vi "Configure Uncaging.vi"(6 "external trigger enabled? (Uncage ONLY)":bool, 7 "Uncage Type":T1, 9 "Gate Waveform (Digital)":digitalwaveform(waveform)={"t0"=timestamp(0 s since 1904-01-01), "dt"=0.0, "Y"={"transitions"=[], "data"=[]}, "error"={"status"=FALSE, "code"=37421928, "source"=""}}, 10 "Pockels Waveform":waveform(dbl), 11 "XY Waveform":waveform(dbl)[](array[waveform])) -> (1 "Gate Task OUT":refnum<k21>, 2 "Pockels Task OUT":refnum<k21>, 3 "XY Mirror voltage Task OUT":refnum<k21>)   [LabVIEW 2012]
uses:
  Custom Controls and Typedefs/UncageType.ctl
  modules/hyperscope modules/hyperscope subVIs/Timebase and Trigger Routing.ctl
  <vilib>/DAQmx/write.llb/DAQmx Write (Analog Wfm 1Chan NSamp).vi
  <vilib>/DAQmx/write.llb/DAQmx Write (Analog 1D Wfm NChan NSamp).vi
  <vilib>/DAQmx/write.llb/DAQmx Write (Digital 1D Wfm NChan NSamp).vi
  GFG/GFGbooleanGet.vi
  <vilib>/DAQmx/create/channels.llb/DAQmx Create Channel (AO-Voltage-Basic).vi
  <vilib>/Waveform/WDTOps.llb/WDT Number of Waveform Samples DBL.vi
  <vilib>/DAQmx/miscellaneous.llb/DAQmx Fill In Error Info.vi
  <vilib>/DAQmx/configure/trigger.llb/DAQmx Start Trigger (Digital Edge).vi
  GFG/GFGstringGet.vi
  <vilib>/DAQmx/create/channels.llb/DAQmx Create Channel (DO-Digital Output).vi
  <vilib>/Waveform/DWDTOps.llb/DWDT Digital Size.vi
  <vilib>/Waveform/DWDTOps.llb/DWDT Uncompress Digital.vi
  <resource>/objmgr/daqmx.rc
  GFG/GFG library.lvlib
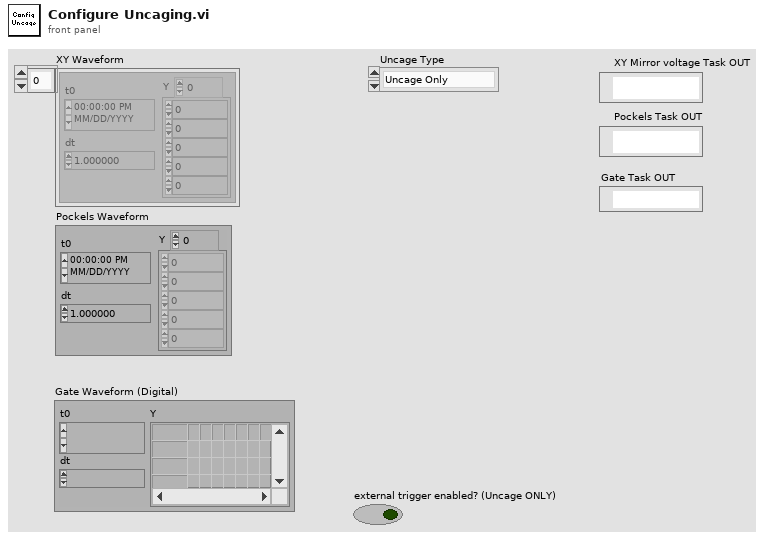
[diagram p1: front panel]
types:
  T1 = typedef "UncageType.ctl" = enum16{"Uncage Only", "Uncage & Image"}
  T2 = typedef "Timebase and Trigger Routing.ctl" = enum16{"Connect", "Disconnect all", "Disconnect Trigger"}
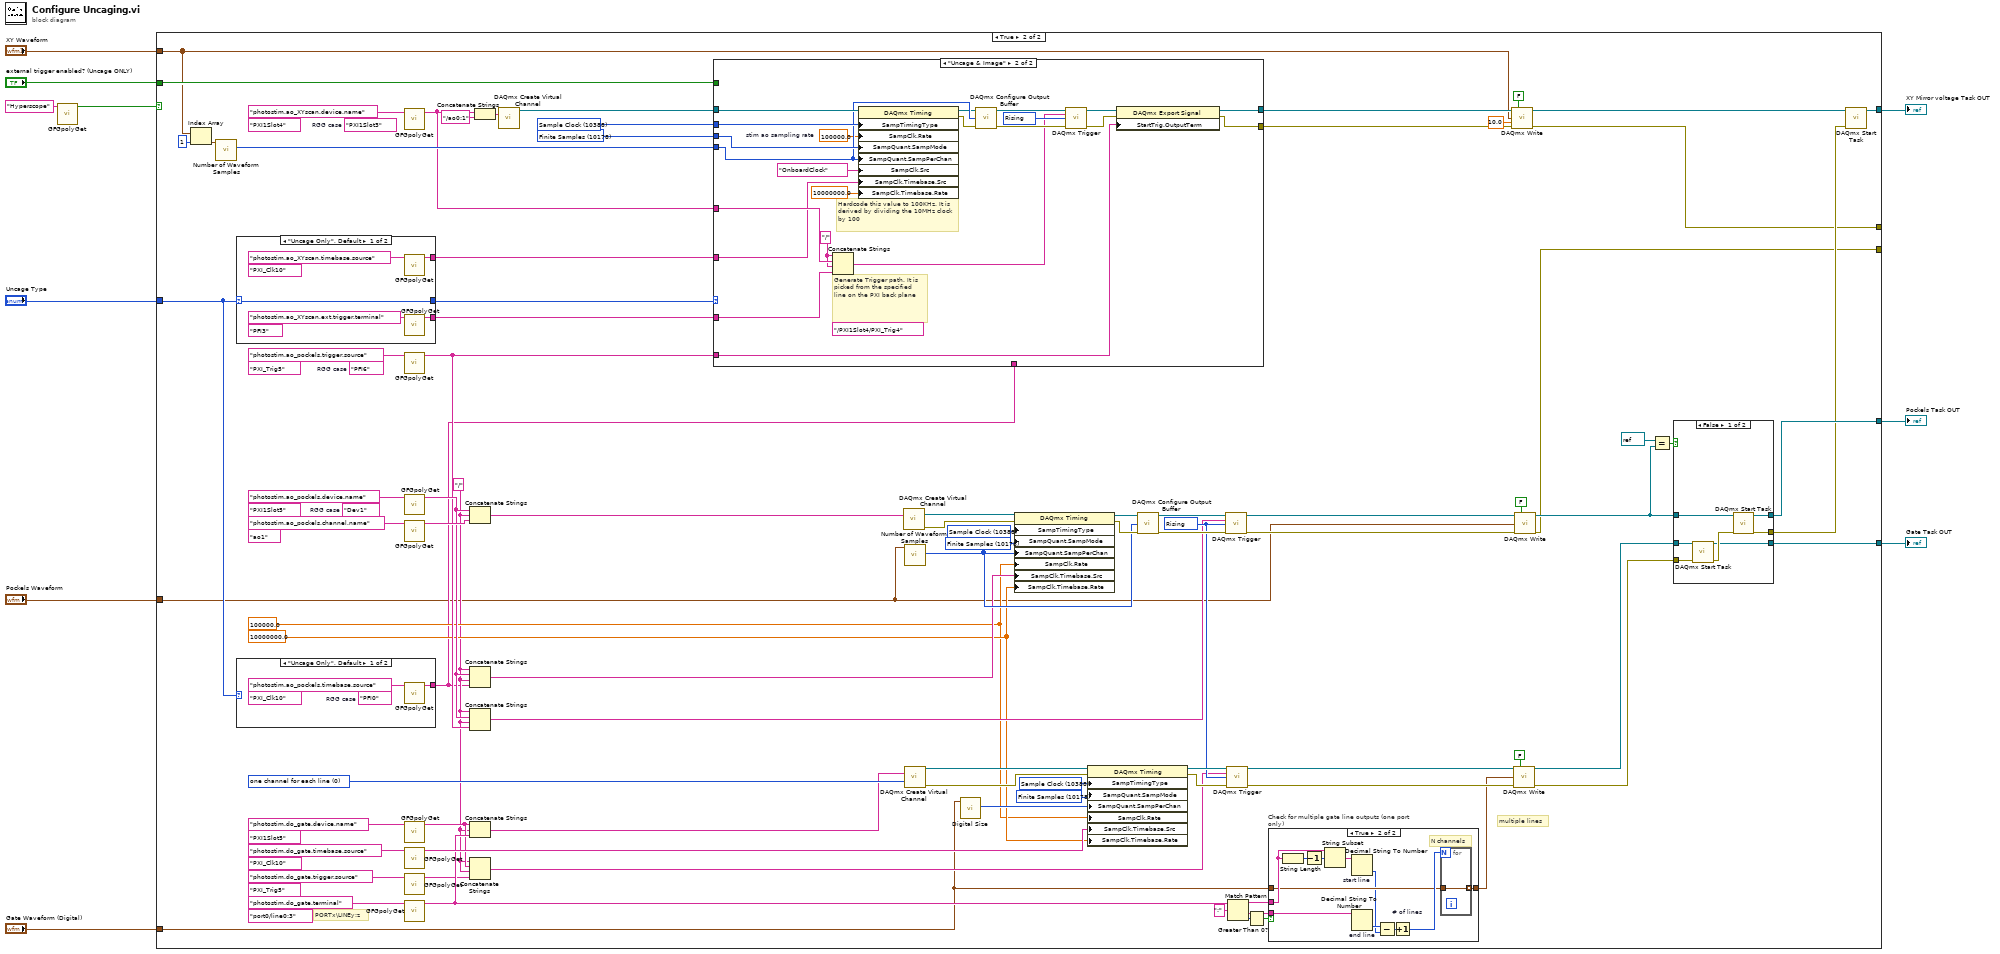
[diagram p0: block diagram]
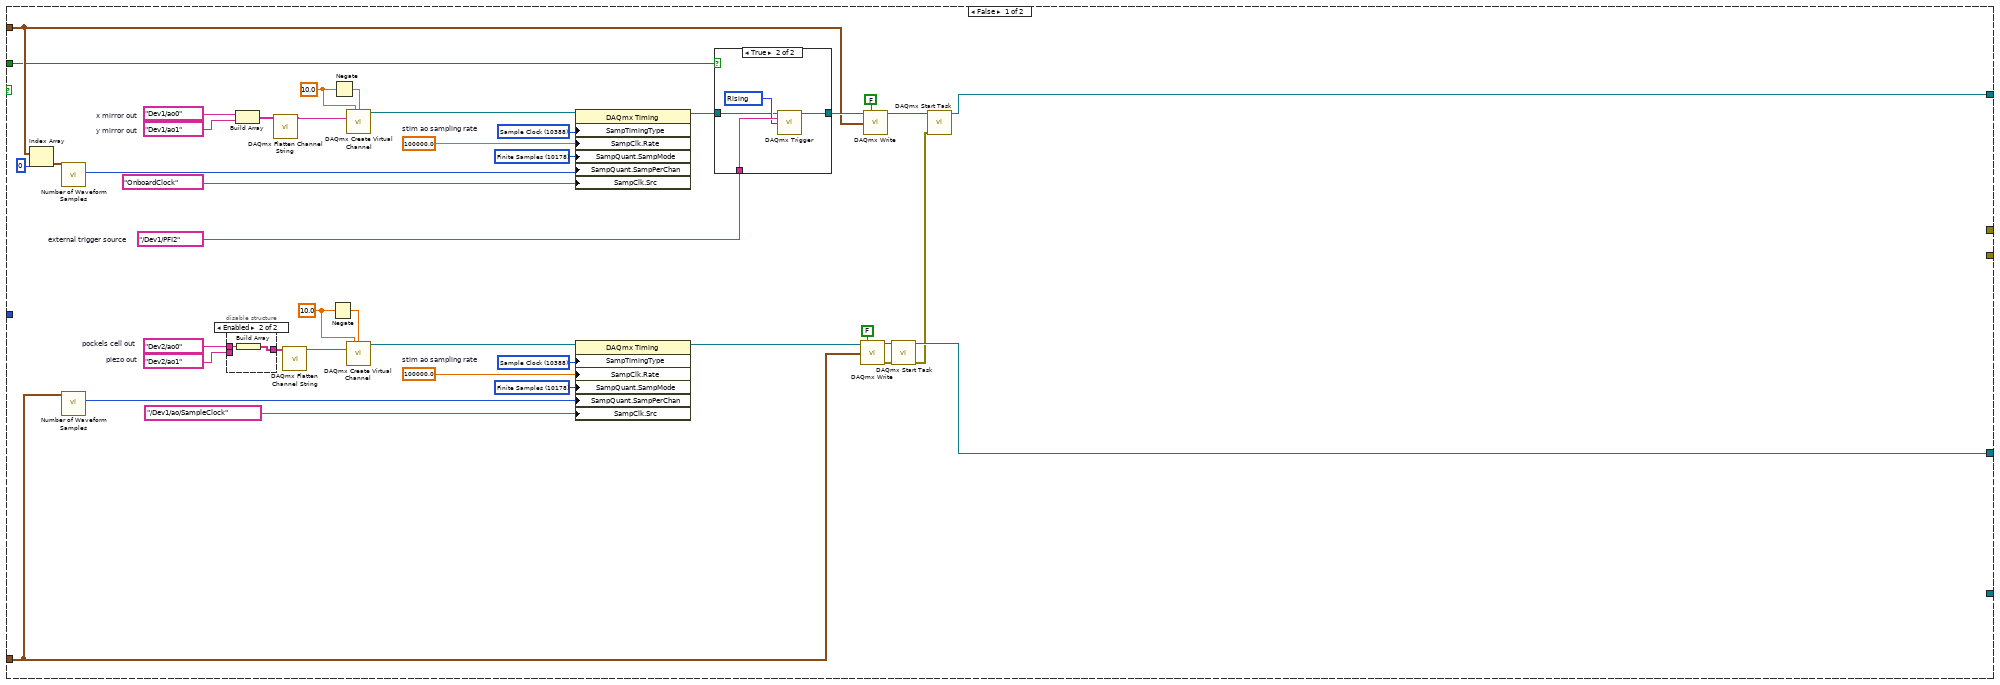
[diagram p2: hidden frame]
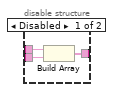
[diagram p3: hidden frame]
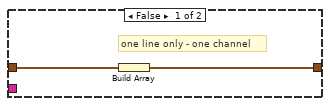
[diagram p5: hidden frame]
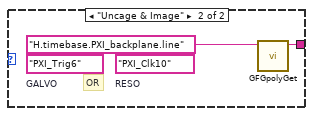
[diagram p6: hidden frame]
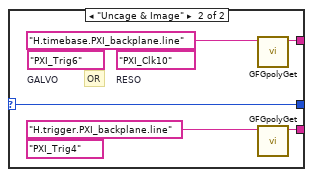
[diagram p7: hidden frame]
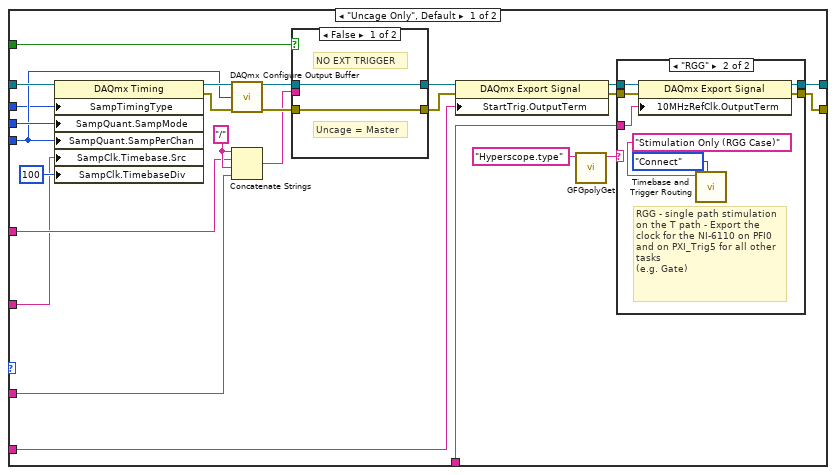
[diagram p8: hidden frame]
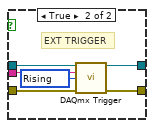
[diagram p10: hidden frame]
diagram:
  n1 = call-poly "GFGpolyGet.vi"("Variable Name in"="Hyperscope") -> ("Boolean Value OUT"=w5:bool)  [unwired: 9 in, 1 out]
  n2 = case shown="True" w5 {
    tunnel: "XY Waveform" -> [w20 w64]
    tunnel: "external trigger enabled? (Uncage ONLY)" -> [w19 w133]
    tunnel: "Uncage Type" -> [_ w121]
    tunnel: [w15 w139] -> w7
    tunnel: [w17 w138] -> w6
    tunnel: "Pockels Waveform" -> [w12 w63]
    tunnel: "Gate Waveform (Digital)" -> [_ w62]
    tunnel: [_ w124] -> w1
    tunnel: [_ w66] -> _
    tunnel: [_ w65] -> _
    frame False {
      w13 = tag "/Dev1/PFI2"  # external trigger source
      w31 = 100000.0  # stim ao sampling rate
      w30 = 100000.0  # stim ao sampling rate
      w37 = 10388 items=["Sample Clock"=10388, "Burst Handshake"=12548, "Handshake"=10389, "Implicit"=10451, "On Demand"=10390, "Change Detection"=12504, "Pipelined Sample Clock"=14668] ("SampTimingType")
      w36 = 10178 items=["Finite Samples"=10178, "Continuous Samples"=10123, "Hardware Timed Single Point"=12522] ("SampQuant.SampMode")
      w38 = 10388 items=["Sample Clock"=10388, "Burst Handshake"=12548, "Handshake"=10389, "Implicit"=10451, "On Demand"=10390, "Change Detection"=12504, "Pipelined Sample Clock"=14668] ("SampTimingType")
      w39 = 10178 items=["Finite Samples"=10178, "Continuous Samples"=10123, "Hardware Timed Single Point"=12522] ("SampQuant.SampMode")
      w42 = 10.0 ("maximum value")
      w44 = 10.0 ("maximum value")
      w46 = tag "Dev2/ao1"  # piezo out
      w47 = tag "Dev2/ao0"  # pockels cell out
      w50 = tag "Dev1/ao1"  # y mirror out
      w51 = tag "Dev1/ao0"  # x mirror out
      n3 = Index Array(array=w20, index=0) -> (element=w23:waveform(dbl))
      n4 = call-poly <vilib>:"Number of Waveform Samples.vi"("waveform in"=w23) -> ("number of samples"=w22:i32)  [unwired: 8 in, 2 out]
      n5 = call-poly <vilib>:"Number of Waveform Samples.vi"("waveform in"=w12) -> ("number of samples"=w21:i32)  [unwired: 8 in, 2 out]
      n6 = disable-structure shown="Enabled" {
        disable-tunnel: [w54 w55] -> w48
        disable-tunnel: w47 -> [w53 w56]
        disable-tunnel: w46 -> [w52 _]
        frame Disabled {
          n7 = Build Array(w53, w52) -> (w54:tag[])
        }
        frame Enabled {
          n8 = Build Array(w56) -> (w55:tag[])
        }
      }
      n9 = Build Array(w51, w50) -> (w49:tag[])
      n10 = call <vilib>:"DAQmx Flatten Channel String.vi"("names in"=w49) -> ("names out"=w43:string)  [unwired: 13 in, 1 out]
      n11 = call <vilib>:"DAQmx Flatten Channel String.vi"("names in"=w48) -> ("names out"=w40:string)  [unwired: 13 in, 1 out]
      n12 = Negate(x=w42) -> (-x=w41:dbl)
      n13 = Negate(x=w44) -> (-x=w45:dbl)
      n14 = call-poly <vilib>:"DAQmx Create Virtual Channel.vi"("maximum value"=w42, "minimum value"=w41, "physical channels"=w40) -> ("task out"=w34:refnum<k21>)  [unwired: 11 in, 1 out]
      n15 = call-poly <vilib>:"DAQmx Create Virtual Channel.vi"("maximum value"=w44, "minimum value"=w45, "physical channels"=w43) -> ("task out"=w35:refnum<k21>)  [unwired: 11 in, 1 out]
      n16 = property class="DAQmx Timing"(reference=w35, "SampTimingType"=w38, "SampClk.Rate"=w30, "SampQuant.SampMode"=w39, "SampQuant.SampPerChan"=w22, "SampClk.Src"=tag "OnboardClock") -> (reference out=w29:refnum<k21>)  [unwired: 1 in, 1 out]
      n17 = property class="DAQmx Timing"(reference=w34, "SampTimingType"=w37, "SampClk.Rate"=w31, "SampQuant.SampMode"=w36, "SampQuant.SampPerChan"=w21, "SampClk.Src"=tag "/Dev1/ao/SampleClock") -> (reference out=w25:refnum<k21>)  [unwired: 1 in, 1 out]
      n18 = case shown="True" w19 {
        tunnel: w13 -> [_ w61]
        tunnel: [w57 w60] -> w27
        tunnel: w29 -> [w57 w58]
        frame False {
        }
        frame True {
          w59 = 10280 items=["Rising"=10280, "Falling"=10171] ("edge")
          n19 = call-poly <vilib>:"DAQmx Trigger.vi"("task/channels in"=w58, "source"=w61, "edge"=w59) -> ("task out"=w60:refnum<k21>)  [unwired: 11 in, 1 out]
        }
      }
      n20 = call-poly <vilib>:"DAQmx Write.vi"("task/channels in"=w25, "auto start"=FALSE, "data"=w12) -> ("task out"=w18:refnum<k21>, "error out"=w11:errorcluster)  [unwired: 10 in, 1 out]
      n21 = call-poly <vilib>:"DAQmx Write.vi"("task/channels in"=w27, "auto start"=FALSE, "data"=w20) -> ("task out"=w16:refnum<k21>)  [unwired: 10 in, 2 out]
      n22 = call <vilib>:"DAQmx Start Task.vi"("task/channels in"=w18, "error in"=w11) -> ("task out"=w17:refnum<k21>, "error out"=w14:errorcluster)  [unwired: 12 in]
      n23 = call <vilib>:"DAQmx Start Task.vi"("task/channels in"=w16, "error in"=w14) -> ("task out"=w15:refnum<k21>)  [unwired: 12 in, 1 out]
    }
    frame True {
      (unwired) tag "Dev1"  # RGG case
      (unwired) tag "PXI1Slot3"  # RGG case
      (unwired) tag "PFI6"  # RGG case
      w69 = 100000.0 ("SampClk.Rate")
      w70 = 10000000.0 ("SampClk.Timebase.Rate")
      (unwired) tag "port0/line0:3" ("lines")
      (unwired) tag "PXI1Slot5" ("lines")
      (unwired) tag "PXI_Trig5" ("physical channels")
      w99 = 0 items=["one channel for each line", "one channel for all lines"] ("line grouping")
      (unwired) tag "PXI_Clk10" ("SampClk.Timebase.Src")
      (unwired) tag "PXI_Trig5" ("source")
      w93 = 10280 items=["Rising"=10280, "Falling"=10171] ("edge")
      w101 = 10178 items=["Finite Samples"=10178, "Continuous Samples"=10123, "Hardware Timed Single Point"=12522] ("SampQuant.SampMode")
      w102 = 10388 items=["Sample Clock"=10388, "Burst Handshake"=12548, "Handshake"=10389, "Implicit"=10451, "On Demand"=10390, "Change Detection"=12504, "Pipelined Sample Clock"=14668] ("SampTimingType")
      (unwired) tag "ao1" ("physical channels")
      w68 = "/" ("string")
      (unwired) tag "PXI1Slot5" ("physical channels")
      w120 = 10388 items=["Sample Clock"=10388, "Burst Handshake"=12548, "Handshake"=10389, "Implicit"=10451, "On Demand"=10390, "Change Detection"=12504, "Pipelined Sample Clock"=14668] ("SampTimingType")
      w119 = 10178 items=["Finite Samples"=10178, "Continuous Samples"=10123, "Hardware Timed Single Point"=12522] ("SampQuant.SampMode")
      (unwired) tag "PXI1Slot4" ("physical channels")
      w148 = 10388 items=["Sample Clock"=10388, "Burst Handshake"=12548, "Handshake"=10389, "Implicit"=10451, "On Demand"=10390, "Change Detection"=12504, "Pipelined Sample Clock"=14668] ("SampTimingType")
      w147 = 10178 items=["Finite Samples"=10178, "Continuous Samples"=10123, "Hardware Timed Single Point"=12522] ("SampQuant.SampMode")
      # "multiple lines"
      # "PORTx\\LINEy:z"
      n24 = Index Array(array=w64, index=1) -> (element=w135:waveform(dbl))
      n25 = call-poly <vilib>:"Number of Waveform Samples.vi"("waveform in"=w135) -> ("number of samples"=w134:i32)  [unwired: 8 in, 2 out]
      n26 = case shown="\"Uncage Only\", Default" w121 {
        selector: w121 -> [w169 w172]
        tunnel: [w171 w176] -> w128
        tunnel: [w167 w175] -> w127
        tunnel: [w169 w172] -> w80
        frame "Uncage Only", Default {
          (unwired) tag "PFI3"
          (unwired) tag "PXI_Clk10" ("SampClk.Timebase.Src")
          n27 = call-poly "GFGpolyGet.vi"("Variable Name in"="photostim.ao_XYscan.timebase.source") -> ("String"=w171:string)  [unwired: 9 in, 1 out]
          n28 = call-poly "GFGpolyGet.vi"("Variable Name in"="photostim.ao_XYscan.ext.trigger.terminal") -> ("String"=w167:string)  [unwired: 9 in, 1 out]
        }
        frame "Uncage & Image" {
          (unwired) tag "PXI_Clk10"  # RESO
          (unwired) tag "PXI_Trig6"  # GALVO
          (unwired) tag "PXI_Trig4" ("physical channels")
          # "OR"
          n29 = call-poly "GFGpolyGet.vi"("Variable Name in"="H.timebase.PXI_backplane.line") -> ("String"=w176:string)  [unwired: 9 in, 1 out]
          n30 = call-poly "GFGpolyGet.vi"("Variable Name in"="H.trigger.PXI_backplane.line") -> ("String"=w175:string)  [unwired: 9 in, 1 out]
        }
      }
      n31 = case shown="\"Uncage Only\", Default" w121 {
        tunnel: [w163 w165] -> w67
        frame "Uncage Only", Default {
          (unwired) tag "PFI0"  # RGG case
          (unwired) tag "PXI_Clk10" ("SampClk.Timebase.Src")
          n32 = call-poly "GFGpolyGet.vi"("Variable Name in"="photostim.ao_pockels.timebase.source") -> ("String"=w163:string)  [unwired: 9 in, 1 out]
        }
        frame "Uncage & Image" {
          (unwired) tag "PXI_Clk10"  # RESO
          (unwired) tag "PXI_Trig6"  # GALVO
          # "OR"
          n33 = call-poly "GFGpolyGet.vi"("Variable Name in"="H.timebase.PXI_backplane.line") -> ("String"=w165:string)  [unwired: 9 in, 1 out]
        }
      }
      n34 = call-poly "GFGpolyGet.vi"("Variable Name in"="photostim.ao_XYscan.device.name") -> ("String"=w129:string)  [unwired: 9 in, 1 out]
      n35 = call-poly "GFGpolyGet.vi"("Variable Name in"="photostim.ao_pockels.trigger.source") -> ("String"=w77:string)  [unwired: 9 in, 1 out]
      n36 = call-poly "GFGpolyGet.vi"("Variable Name in"="photostim.ao_pockels.device.name") -> ("String"=w104:string)  [unwired: 9 in, 1 out]
      n37 = call-poly "GFGpolyGet.vi"("Variable Name in"="photostim.ao_pockels.channel.name") -> ("String"=w111:string)  [unwired: 9 in, 1 out]
      n38 = call-poly "GFGpolyGet.vi"("Variable Name in"="photostim.do_gate.device.name") -> ("String"=w74:string)  [unwired: 9 in, 1 out]
      n39 = call-poly "GFGpolyGet.vi"("Variable Name in"="photostim.do_gate.timebase.source") -> ("String"=w90:string)  [unwired: 9 in, 1 out]
      n40 = call-poly "GFGpolyGet.vi"("Variable Name in"="photostim.do_gate.trigger.source") -> ("String"=w73:string)  [unwired: 9 in, 1 out]
      n41 = call-poly "GFGpolyGet.vi"("Variable Name in"="photostim.do_gate.terminal") -> ("String"=w82:string)  [unwired: 9 in, 1 out]
      n42 = Concatenate Strings(w104, w68, w111) -> (w110:string)
      n43 = Concatenate Strings(w68, w104, w68, w67) -> (w89:string)
      n44 = Concatenate Strings(w68, w104, w68, w77) -> (w78:string)
      n45 = Concatenate Strings(w74, w68, w82) -> (w88:string)
      n46 = Concatenate Strings(w68, w74, w68, w73) -> (w72:string)
      n47 = Concatenate Strings(w129, "/ao0:1" ("string")) -> (w130:string)
      n48 = call-poly <vilib>:"DAQmx Create Virtual Channel.vi"("physical channels"=w130) -> ("task out"=w136:refnum<k21>)  [unwired: 13 in, 1 out]
      n49 = case shown="\"Uncage & Image\"" w80 {
        tunnel: w148 -> [w190 w240]
        tunnel: w147 -> [w201 w239]
        tunnel: [w180 w237] -> w122
        tunnel: w136 -> [w200 w238]
        tunnel: w134 -> [w198 w236]
        tunnel: w133 -> [w196 _]
        tunnel: [w179 w235] -> w123
        tunnel: w129 -> [w189 w234]
        tunnel: w128 -> [w185 w233]
        tunnel: w127 -> [w183 w232]
        tunnel: w77 -> [w184 w231]
        tunnel: w67 -> [w177 _]
        frame "Uncage Only", Default {
          w192 = "/" ("string")
          n50 = property class="DAQmx Timing"(reference=w200, "SampTimingType"=w190, "SampQuant.SampMode"=w201, "SampQuant.SampPerChan"=w198, "SampClk.Timebase.Src"=w185, "SampClk.TimebaseDiv"=u32 100) -> (reference out=w199:refnum<k21>, error out=w194:errorcluster)  [unwired: 1 in]
          n51 = call <vilib>:"DAQmx Configure Output Buffer.vi"("task/channels in"=w199, "buffer size (in samples per channel)"=w198, "error in"=w194) -> ("task out"=w197:refnum<k21>, "error out"=w193:errorcluster)  [unwired: 11 in]
          n52 = Concatenate Strings(w192, w189, w192, w183) -> (w191:string)
          n53 = case shown="False" w196 {
            tunnel: w191 -> [_ w218]
            tunnel: [w212 w217] -> w187
            tunnel: w197 -> [w212 w215]
            tunnel: w193 -> [w211 w214]
            tunnel: [w211 w213] -> w188
            frame False {
              # "Uncage = Master"
              # "NO EXT TRIGGER"
            }
            frame True {
              w216 = 10280 items=["Rising"=10280, "Falling"=10171] ("edge")
              # "EXT TRIGGER"
              n54 = call-poly <vilib>:"DAQmx Trigger.vi"("task/channels in"=w215, "source"=w218, "edge"=w216, "error in"=w214) -> ("task out"=w217:refnum<k21>, "error out"=w213:errorcluster)  [unwired: 10 in]
            }
          }
          n55 = property class="DAQmx Export Signal"(reference=w187, error in=w188, "StartTrig.OutputTerm"=w184) -> (reference out=w182:refnum<k21>, error out=w181:errorcluster)
          n56 = call-poly "GFGpolyGet.vi"("Variable Name in"="Hyperscope.type") -> ("String"=w178:string)  [unwired: 9 in, 1 out]
          n57 = case shown="\"RGG\"" w178 {
            tunnel: w182 -> [w203 w210]
            tunnel: w181 -> [w202 w209]
            tunnel: [w203 w208] -> w180
            tunnel: [w202 w207] -> w179
            tunnel: w177 -> [_ w206]
            frame Default {
            }
            frame "RGG" {
              # "RGG - single path stimulation on the T path - Export the clock for the NI-6110 on PFI0 and on PXI_Trig5 for all other tasks\n(e.g. Gate)"
              n58 = property class="DAQmx Export Signal"(reference=w210, error in=w209, "10MHzRefClk.OutputTerm"=w206) -> (reference out=w208:refnum<k21>, error out=w207:errorcluster)
              n59 = call "Timebase and Trigger Routing.vi"("Signal Router Action"=Timebase_and_Trigger_Routing."Connect", "System Type"="Stimulation Only (RGG Case)" ("Variable Name in")) -> ()  [unwired: 9 in, 1 out]
            }
          }
        }
        frame "Uncage & Image" {
          w223 = 100000.0  # stim ao sampling rate
          w225 = "/" ("string")
          (unwired) tag "/PXI1Slot4/PXI_Trig4" ("source")
          w230 = 10280 items=["Rising"=10280, "Falling"=10171] ("edge")
          # "Generate Trigger path. It is picked from the specified line on the PXI back plane"
          # "Hardcode this value to 100KHz. It is derived by dividing the 10MHz clock by 100"
          n60 = Concatenate Strings(w225, w234, w225, w232) -> (w224:string)
          n61 = property class="DAQmx Timing"(reference=w238, "SampTimingType"=w240, "SampClk.Rate"=w223, "SampQuant.SampMode"=w239, "SampQuant.SampPerChan"=w236, "SampClk.Src"=tag "OnboardClock", "SampClk.Timebase.Src"=w233, "SampClk.Timebase.Rate"=10000000.0) -> (reference out=w228:refnum<k21>, error out=w227:errorcluster)  [unwired: 1 in]
          n62 = call <vilib>:"DAQmx Configure Output Buffer.vi"("task/channels in"=w228, "buffer size (in samples per channel)"=w236, "error in"=w227) -> ("task out"=w229:refnum<k21>, "error out"=w226:errorcluster)  [unwired: 11 in]
          n63 = call-poly <vilib>:"DAQmx Trigger.vi"("task/channels in"=w229, "source"=w224, "edge"=w230, "error in"=w226) -> ("task out"=w220:refnum<k21>, "error out"=w221:errorcluster)  [unwired: 10 in]
          n64 = property class="DAQmx Export Signal"(reference=w220, error in=w221, "StartTrig.OutputTerm"=w231) -> (reference out=w237:refnum<k21>, error out=w235:errorcluster)
        }
      }
      n65 = call-poly <vilib>:"DAQmx Create Virtual Channel.vi"("physical channels"=w110) -> ("task out"=w118:refnum<k21>, "error out"=w114:errorcluster)  [unwired: 13 in]
      n66 = call-poly <vilib>:"Number of Waveform Samples.vi"("waveform in"=w63) -> ("number of samples"=w108:i32)  [unwired: 8 in, 2 out]
      n67 = call-poly <vilib>:"DAQmx Create Virtual Channel.vi"("lines"=w88, "line grouping"=w99) -> ("task out"=w103:refnum<k21>, "error out"=w98:errorcluster)  [unwired: 12 in]
      n68 = call-poly <vilib>:"Digital Size.vi"("digital waveform in"=w62) -> ("number of samples"=w100:i32)  [unwired: 7 in, 3 out]
      n69 = property class="DAQmx Timing"(reference=w118, error in=w114, "SampTimingType"=w120, "SampQuant.SampMode"=w119, "SampQuant.SampPerChan"=w108, "SampClk.Rate"=w69, "SampClk.Timebase.Src"=w89, "SampClk.Timebase.Rate"=w70) -> (reference out=w107:refnum<k21>, error out=w109:errorcluster)
      n70 = property class="DAQmx Timing"(reference=w103, error in=w98, "SampTimingType"=w102, "SampQuant.SampMode"=w101, "SampQuant.SampPerChan"=w100, "SampClk.Rate"=w69, "SampClk.Timebase.Src"=w90, "SampClk.Timebase.Rate"=w70) -> (reference out=w97:refnum<k21>, error out=w96:errorcluster)
      n71 = call <vilib>:"DAQmx Configure Output Buffer.vi"("task/channels in"=w107, "buffer size (in samples per channel)"=w108, "error in"=w109) -> ("task out"=w106:refnum<k21>, "error out"=w105:errorcluster)  [unwired: 11 in]
      n72 = call-poly <vilib>:"DAQmx Trigger.vi"("task/channels in"=w106, "source"=w78, "edge"=w93, "error in"=w105) -> ("task out"=w116:refnum<k21>, "error out"=w115:errorcluster)  [unwired: 10 in]
      n73 = call-poly <vilib>:"DAQmx Trigger.vi"("task/channels in"=w97, "source"=w72, "edge"=w93, "error in"=w96) -> ("task out"=w94:refnum<k21>, "error out"=w95:errorcluster)  [unwired: 10 in]
      n74 = Match Pattern(string=w82, regular expression=":") -> (before substring=w83:string, after substring=w84:string, offset past match=w86:i32)  [unwired: 1 in, 1 out]
      n75 = Greater Than 0?(x=w86) -> (x > 0?=w85:bool)
      n76 = case "Check for multiple gate line outputs (one port only)" shown="True" w85 {
        tunnel: w84 -> [_ w161]
        tunnel: w83 -> [_ w158]
        tunnel: w62 -> [w150 w153]
        tunnel: [w149 w152] -> w81
        frame False {
          # "one line only - one channel"
          n77 = Build Array(w150) -> (w149:digitalwaveform[])
        }
        frame True {
          # "N channels"
          n78 = String Length(string=w158) -> (length=w159:i32)
          n79 = Decrement(x=w159) -> (x-1=w160:i32)
          n80 = String Subset(string=w158, offset (0)=w160) -> (substring=w157:string)  [unwired: 1 in]
          n81 = Decimal String To Number "start line"(string=w157) -> (number=w151:i32)  [unwired: 2 in, 1 out]
          n82 = Decimal String To Number "end line"(string=w161) -> (number=w156:i32)  [unwired: 2 in, 1 out]
          n83 = Subtract(x=w156, y=w151) -> (x-y=w155:i32)
          n84 = Increment "# of lines"(x=w155) -> (x+1=w154:i32)
          n85 = for {
            N: w154 -> [_]
            tunnel: w153 -> [w162]
            tunnel: [w162] -> w152 mode=indexing
          }
        }
      }
      n86 = call-poly <vilib>:"DAQmx Write.vi"("task/channels in"=w122, "auto start"=FALSE, "data"=w64, "timeout"=10.0, "error in"=w123) -> ("task out"=w140:refnum<k21>, "error out"=w66:errorcluster)  [unwired: 8 in, 1 out]
      n87 = call-poly <vilib>:"DAQmx Write.vi"("task/channels in"=w94, "auto start"=FALSE, "data"=w81, "error in"=w95) -> ("task out"=w125:refnum<k21>, "error out"=w126:errorcluster)  [unwired: 9 in, 1 out]
      n88 = call-poly <vilib>:"DAQmx Write.vi"("task/channels in"=w116, "auto start"=FALSE, "data"=w63, "error in"=w115) -> ("task out"=w141:refnum<k21>, "error out"=w65:errorcluster)  [unwired: 9 in, 1 out]
      n89 = Equal?(x=refnum<k21> refnum ("task out"), y=w141) -> (x = y?=w142:bool)
      n90 = case shown="False" w142 {
        tunnel: w141 -> [w247 w249]
        tunnel: [w246 w249] -> w138
        tunnel: [w245 _] -> w137
        tunnel: w126 -> [w243 _]
        tunnel: w125 -> [w242 w248]
        tunnel: [w241 w248] -> w124
        frame False {
          n91 = call <vilib>:"DAQmx Start Task.vi"("task/channels in"=w242, "error in"=w243) -> ("task out"=w241:refnum<k21>, "error out"=w244:errorcluster)  [unwired: 12 in]
          n92 = call <vilib>:"DAQmx Start Task.vi"("task/channels in"=w247, "error in"=w244) -> ("task out"=w246:refnum<k21>, "error out"=w245:errorcluster)  [unwired: 12 in]
        }
        frame True {
        }
      }
      n93 = call <vilib>:"DAQmx Start Task.vi"("task/channels in"=w140, "error in"=w137) -> ("task out"=w139:refnum<k21>)  [unwired: 12 in, 1 out]
    }
  }
  "XY Mirror voltage Task OUT" <- w7
  "Pockels Task OUT" <- w6
  "Gate Task OUT" <- w1
